vi "Thread Parameters.Get Processor.vi"(11 "Thread Parameters in":refnum<class "Thread Parameters.lvclass">) -> (2 "Processor":i32=-2, 3 "Thread Parameters out":refnum<class "Thread Parameters.lvclass">)   [LabVIEW 2016, in "DSF.Engine.lvlib" / "Thread Parameters.lvclass"]
uses:
  Thread Parameters.lvclass
  Thread Parameters.lvclass/Thread Parameters.ctl
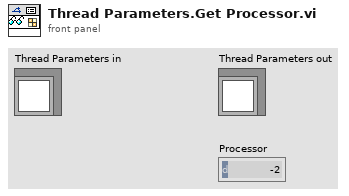
[diagram p1: front panel]
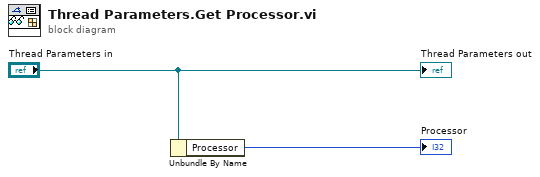
[diagram p0: block diagram]
diagram:
  n1 = Unbundle By Name("Thread Parameters in") -> ("Processor"=→"Processor":i32)
  "Thread Parameters out" <- "Thread Parameters in"
